vi "Prepare Save Dir.vi"(9 "Entity Extension (\".lvclass\")":string=".lvclass", 10 "Entity Name":string, 11 "Owning LVLib":refnum<vi>) -> (1 "Entity Path":path, 3 "Owning LVLib Dup":refnum<vi>)   [LabVIEW 2013]
doc: "Copyright (c) 2016 Sze Howe Koh\n\nThis Source Code Form is subject to the terms of the Mozilla Public License, v. 2.0. If a copy of the MPL was not distributed with this file, You can obtain one at http://mozilla.org/MPL/2.0/."
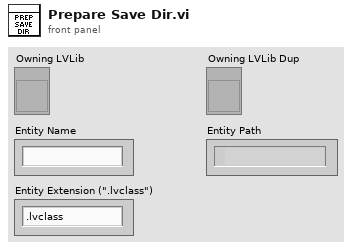
[diagram p1: front panel]
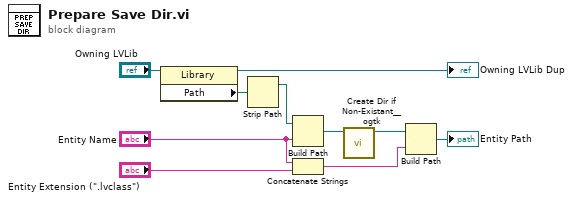
[diagram p0: block diagram]
diagram:
  n1 = property class="Library"(reference="Owning LVLib") -> (reference out=→"Owning LVLib Dup":refnum<vi>, "Path"=w3:path)  [unwired: 1 in, 1 out]
  n2 = Strip Path(path=w3) -> (stripped path=w2:path)  [unwired: 1 out]
  n3 = Build Path(base path=w2, name or relative path="Entity Name") -> (appended path=w9:path)
  n4 = Concatenate Strings("Entity Name", "Entity Extension (\".lvclass\")") -> (w6:string)
  n5 = call <userlib>:"Create Dir if Non-Existant__ogtk.vi"("Directory Path"=w9) -> ("dup Directory Path"=w10:path)  [unwired: 8 in, 2 out]
  n6 = Build Path(base path=w10, name or relative path=w6) -> (appended path=→"Entity Path":path)
